vi "Setup UI.vi"(8 "error in (no error)":errorcluster, 10 "Set UI to input? (F)":bool, 11 "Lockin and Fluke Multimeter in":refnum<class "Lockin and Fluke Multimeter.lvclass">) -> (0 "error out":errorcluster, 3 "Lockin and Fluke Multimeter out":refnum<class "Lockin and Fluke Multimeter.lvclass">)   [LabVIEW 2017, in "Lockin and Fluke Multimeter.lvclass"]
doc: "Setup UI constructs an object -- populates its member fields -- from a front panel the user can see. The VI should be as simple as possible so that a UI loop can poll it continuously for updates. \n\nThe VI is designed to be used as a subPanel within another VI. Wire true to \"Set UI to input\" only on the first call, just after inserting this VI into a subPanel, to populate its controls with the class's current values.\n\nSetup UI is distinct from the class constructor. Class constructors are not polymorphic, yet configure dialogs need to configure objects without knowing their type -- and polymorphism is the necessary solution. Thus, Setup UI is a polymorphic class constructor. This continously polled \"Setup UI\" concept is a kludge: a better idea would be an XControl, but those require a steeper learning curve."
uses:
  Lockin and Fluke Multimeter.lvclass
  Lockin/Sensitivity.ctl
  Lockin and Fluke Multimeter.lvclass/Lockin and Fluke Multimeter.ctl
  Utility Classes/Readable/Readable.lvclass
  Lockin/sr830/SR830.lvlib
  Lockin/Lockin SR830.lvclass
panel:
  in  "Lockin multiplier":dbl=1.0
  in  "Ratio multiplier":dbl=1.0
  in  "Fluke multiplier":dbl=1.0
  out "trigger mode (0:internal)":u16(ring) items=["internal - continuous trigger", "external - rear panel trigger with delay", "external - bus trigger with delay", "external - rear panel trigger", "external - bus trigger"]
  in  "rate (0:slow)":u16(ring) items=["slow", "medium", "fast"]
  in  "range (0:auto)":u16(ring) items=["autorange", "200mV, 200 ohms", "2V, 2 kohms", "20V, 20 kohms", "200V, 200 kohms", "1000Vdc, 700 Vac, 2 Mohms", "20 Mohms"]
  out "function (0:volts DC)":u16(ring) items=["volts DC", "volts AC", "2-wire k.ohms", "4-wire k.ohms", "mA DC", "mA AC"]
  in  "Set SR830 tau & sens":bool
  in  "Tau":u16(ring) items=["10 us", "30 us", "100 us", "300 us", "1 ms", "3 ms", "10 ms", "30 ms", "100 ms", "300 ms", "1 s", "3 s", "10 s", "30 s", "100 s", "300 s", "1 ks", "3 ks", "10 ks", "30 ks"]
  in  "Sensitivity":T1 items=["2 nV", "5 nV", "10 nV", "20 nV", "50 nV", "100 nV", "200 nV", "500 nV", "1 uV", "2 uV", "5 uV", "10 uV", "20 uV", "50 uV", "100 uV", "200 uV", "500 uV", "1 mV", "2 mV", "5 mV", "10 mV", "20 mV", "50 mV", "100 mV", "200 mV", "500 mV", "1 V"]
  out "Reference mode":enum16{"external", "internal"}(ring)
  out "Frequency":dbl[unit]
  # "Lockin & Fluke Reader Setup"
  # "Fluke multimeter 3 (GPIB 15)"
  # "SR830"
  # "Fluke changes will be implemented during the \"Read\" action"
  # "This plots & outputs 5 columns:\nSR830: (X, Y, R) * (Lockin multiplier)\nFluke = Fluke output * (Fluke multiplier)\nRatio = X/(Fluke output) * (Ratio mult)\n\n(Plot & output must be the same.)"
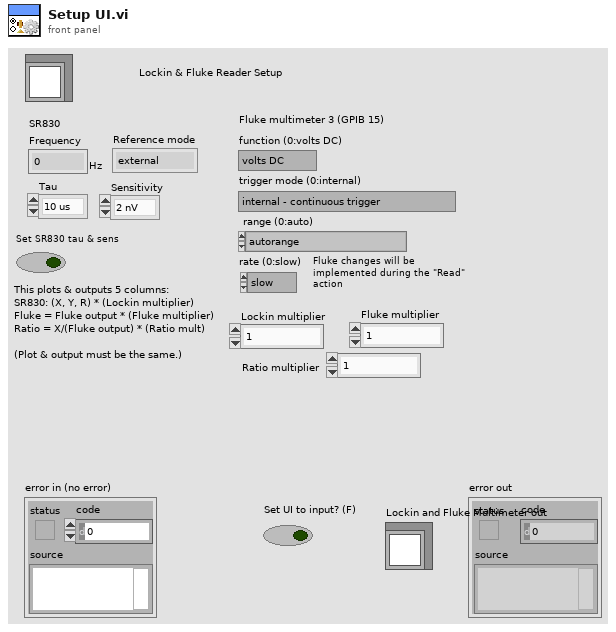
[diagram p1: front panel]
types:
  T1 = typedef "Lockin SR830.lvclass/Sensitivity.ctl" = u16
  T2 = typedef "SR830.lvlib/Tau.ctl" = u16
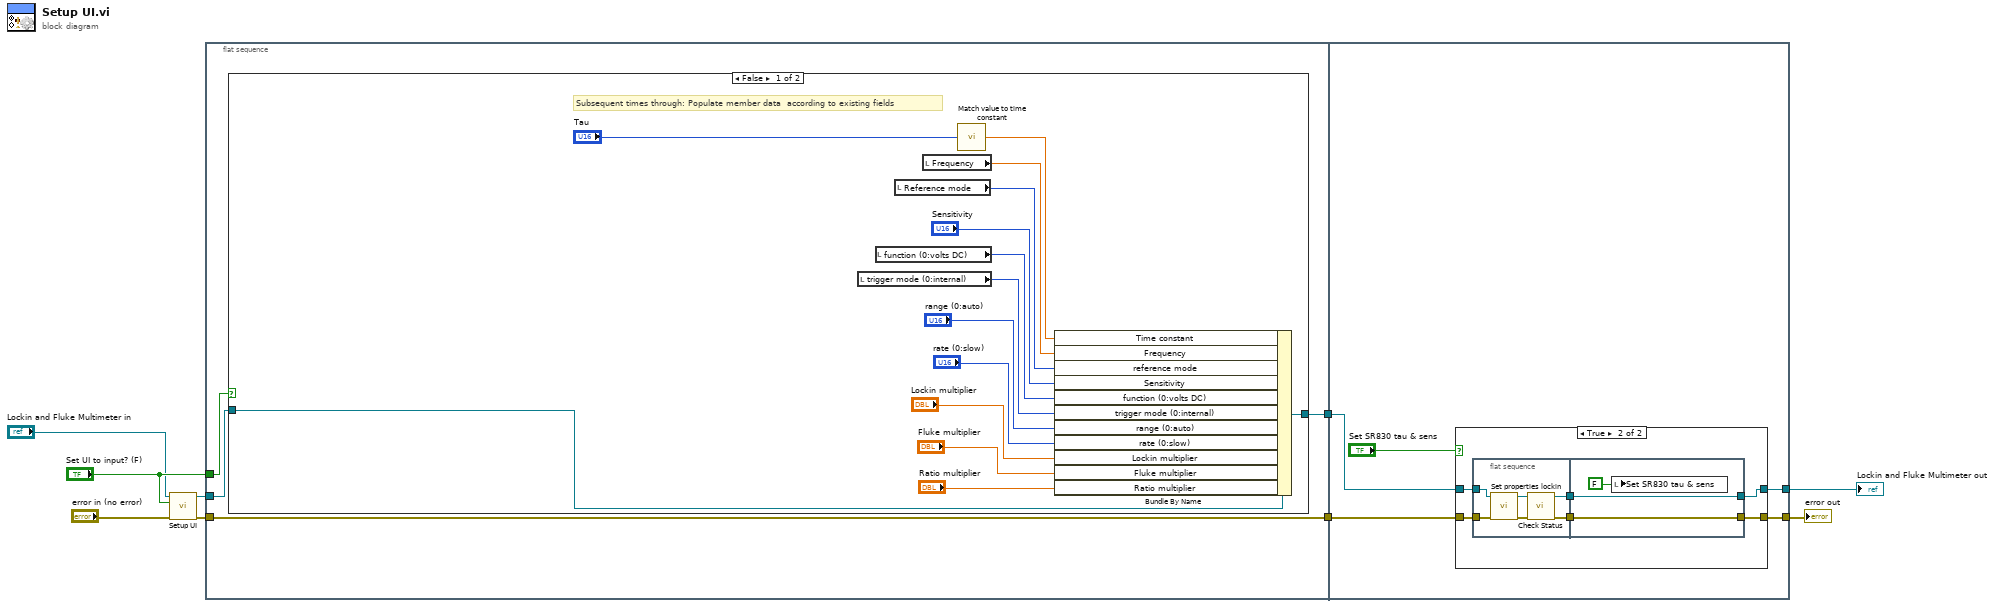
[diagram p0: block diagram]
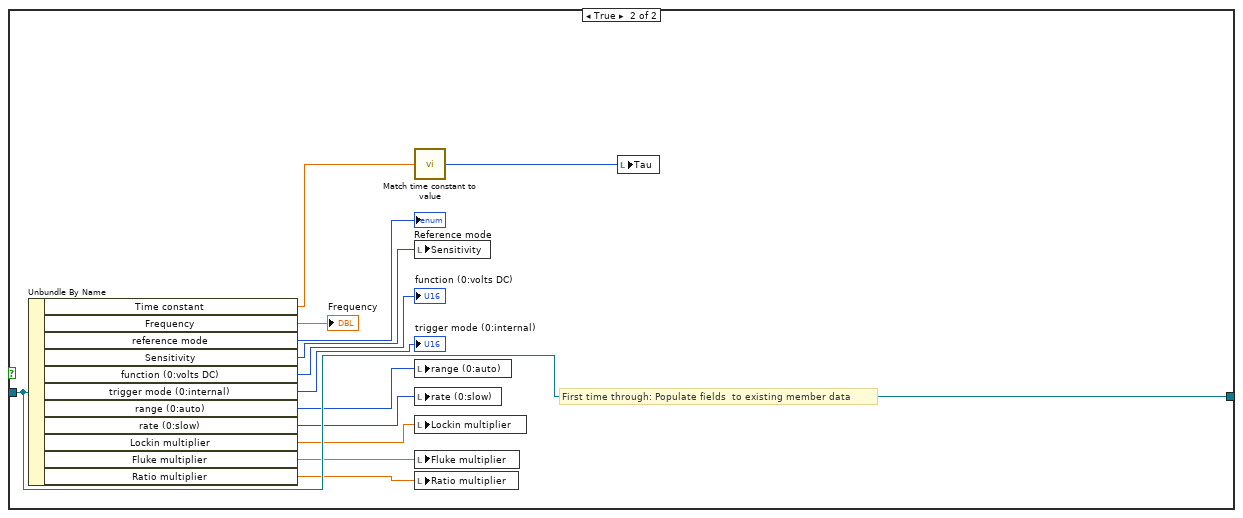
[diagram p2: hidden frame]
diagram:
  n1 = call-parent "Setup UI.vi"("error in (no error)"="error in (no error)", "Set UI to input? (F)"="Set UI to input? (F)", "Instrument in"="Lockin and Fluke Multimeter in") -> ("error out"=w4:errorcluster, "Instrument out"=w7:refnum<class "Lockin and Fluke Multimeter.lvclass">)  [unwired: 7 in]
  n2 = flat-sequence {
    tunnel: "Set UI to input? (F)" -> [w13]
    tunnel: w7 -> [w12]
    tunnel: [w11] -> w6
    tunnel: [w10] -> w5
    tunnel: w4 -> [w10]
    tunnel: w6 -> [w43]
    tunnel: w5 -> [w44]
    tunnel: [w42] -> w3
    tunnel: [w41] -> w2
    frame #0 {
      n3 = case shown="False" w13 {
        tunnel: w12 -> [w27 w37]
        tunnel: [w23 w37] -> w11
        frame False {
          # "Subsequent times through: Populate member data  according to existing fields"
          n4 = local read "trigger mode (0:internal)"() -> (w18:u16)
          n5 = local read "function (0:volts DC)"() -> (w17:u16)
          n6 = local read "Reference mode"() -> (w22:enum16{"external", "internal"})
          n7 = local read "Frequency"() -> (w21:dbl[unit])
          n8 = call "Match value to time constant.vi"("Tau"="Tau") -> ("time constant"=w25:dbl[unit])
          n9 = Bundle By Name(cluster=w27, "Time constant"=w25, "Frequency"=w21, "reference mode"=w22, "Sensitivity"="Sensitivity", "function (0:volts DC)"=w17, "trigger mode (0:internal)"=w18, "range (0:auto)"="range (0:auto)", "rate (0:slow)"="rate (0:slow)", "Lockin multiplier"="Lockin multiplier", "Fluke multiplier"="Fluke multiplier", "Ratio multiplier"="Ratio multiplier") -> (w23:refnum<class "Lockin and Fluke Multimeter.lvclass">)
        }
        frame True {
          # "First time through: Populate fields  to existing member data"
          n10 = Unbundle By Name(w37) -> ("Time constant"=w40:dbl[unit], "Frequency"=→"Frequency":dbl[unit], "reference mode"=→"Reference mode":enum16{"external", "internal"}, "Sensitivity"=w38:T1, "function (0:volts DC)"=→"function (0:volts DC)":u16, "trigger mode (0:internal)"=→"trigger mode (0:internal)":u16, "range (0:auto)"=w35:u16, "rate (0:slow)"=w36:u16, "Lockin multiplier"=w30:dbl, "Fluke multiplier"=w29:dbl, "Ratio multiplier"=w28:dbl)
          n11 = call "Match time constant to value.vi"("Time constant"=w40) -> ("Tau"=w39:T2)
          n12 = local write "Sensitivity"(w38) -> ()
          n13 = local write "range (0:auto)"(w35) -> ()
          n14 = local write "rate (0:slow)"(w36) -> ()
          n15 = local write "Lockin multiplier"(w30) -> ()
          n16 = local write "Fluke multiplier"(w29) -> ()
          n17 = local write "Ratio multiplier"(w28) -> ()
          n18 = local write "Tau"(w39) -> ()
        }
      }
    }
    frame #1 {
      n19 = case shown="True" "Set SR830 tau & sens" {
        tunnel: w44 -> [w46 w53]
        tunnel: w43 -> [w47 w52]
        tunnel: [w47 w50] -> w42
        tunnel: [w46 w49] -> w41
        frame False {
        }
        frame True {
          n20 = flat-sequence {
            tunnel: w53 -> [w57]
            tunnel: w52 -> [w56]
            tunnel: [w55] -> w51
            tunnel: [w54] -> w48
            tunnel: w51 -> [w61]
            tunnel: [w61] -> w50
            tunnel: [w60] -> w49
            tunnel: w48 -> [w60]
            frame #0 {
              n21 = call "Set properties lockin.vi"("error in (no error)"=w57, "Lockin and Fluke Multimeter in"=w56) -> ("error out"=w58:errorcluster, "Lockin and Fluke Multimeter out"=w59:refnum<class "Lockin and Fluke Multimeter.lvclass">)  [unwired: 8 in]
              n22 = call-dynamic "Check Status.vi"("error in (no error)"=w58, "Lockin and Fluke Multimeter in"=w59) -> ("error out"=w54:errorcluster, "Lockin and Fluke Multimeter out"=w55:refnum<class "Lockin and Fluke Multimeter.lvclass">)  [unwired: 6 in, 2 out]
            }
            frame #1 {
              n23 = local write "Set SR830 tau & sens"(FALSE ("Set Parameters")) -> ()
            }
          }
        }
      }
    }
  }
  "error out" <- w2
  "Lockin and Fluke Multimeter out" <- w3
